vi "uService GUI.vi"(8 "error in (no error)":errorcluster, 11 "uService Template in":refnum<class "Tamer.lvclass">) -> (3 "uService Template out":refnum<class "Tamer.lvclass">)   [LabVIEW 2020, in "CIRCUS_uServices.lvlib" / "Tamer.lvlib" / "Tamer.lvclass"]
uses:
  Tamer.lvclass
  Tamer.lvclass/Tamer.ctl
  Link Chain GUI.ctl
  Monkey Summary.ctl
  TALOS/TALOS_PPL.lvlibp/Father of all uServices/Father of all uServices/Father of all uServices.lvclass
  TALOS/TALOS_PPL.lvlibp
  TALOS/TALOS_PPL.lvlibp/Guardian/Guardian/Requests.ctl
  TALOS/TALOS_PPL.lvlibp/Guardian/Guardian/Guardian.lvclass
  Run Utilities/TypeDefs/Monkey Status.ctl
  Run Utilities/Run Utilities.lvlib
  Stop Message.ctl
  C:/Users/marco/Documents/GitHub_Lab/CIRCUS/TALOS/TALOS_PPL.lvlibp/Father of all uServices/Father of all uServices/Father of all uServices.lvclass
  C:/Users/marco/Documents/GitHub_Lab/CIRCUS/TALOS/TALOS_PPL.lvlibp/Ancestor/Ancestor/Ancestor.lvclass
  C:/Users/marco/Documents/GitHub_Lab/CIRCUS/TALOS/Actor Framework.lvlibp/1abvi3w/vi.lib/ActorFramework/Actor/Actor.lvclass
  C:/Users/marco/Documents/GitHub_Lab/CIRCUS/CIRCUS uServices et al/Tamer/Tamer.lvclass
  Monkeys on display - picture.ctl
panel:
  in  "Pause":bool
  in  "Gracefully":bool=TRUE
  in  "Kill Process":bool
  in  "Skip Run":bool
  in  "Monkeys on display":T1
  in  "Tamer Picture":picture
  in  "Color 5":u32(colorbox)=16711680
  in  "Color 4":u32(colorbox)=8454019
  in  "Color 3":u32(colorbox)=16580480
  in  "Color 2":u32(colorbox)=8437759
  in  "Color":u32(colorbox)=16777225
  in  "Debug Mode":bool caption="Open the Debug\nWindow"
  out "Action History":string
  in  "Process":string(combo)
  out "The Stage":T2[][](array[typedef])
  in  "Rerun":bool
  in  "Stop Schedule":bool
  in  "stop New uService":bool
  in  "Reschedule":bool
  in  "Tamer Logo":picture
  # "The TAMER"
  # "Legend:"
  # "Stopped by an error"
  # "Finished well"
  # "Stopped by a user"
  # "Working"
  # "Pre-run init"
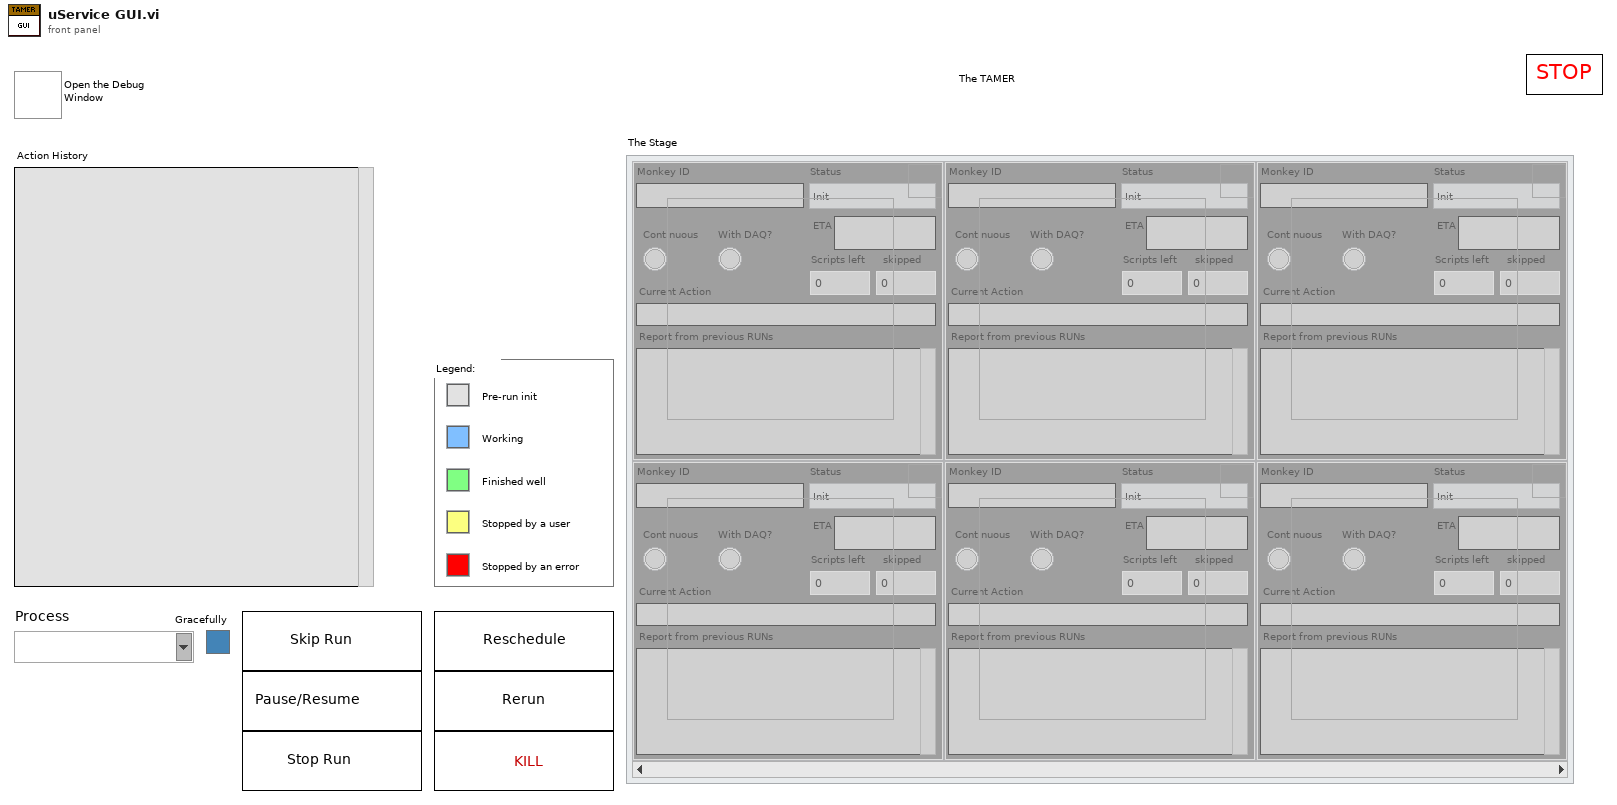
[diagram p1: front panel]
types:
  T1 = typedef "CIRCUS_uServices.lvlib/Tamer.lvlib/Tamer.lvclass/Monkeys on display - picture.ctl" = u16
  T2 = typedef "CIRCUS_uServices.lvlib/Tamer.lvlib/Tamer.lvclass/Monkey Summary.ctl" = cluster{"Color":u32, "Status":T3, "Continuous":bool, "Scripts left":u32, "Scripts skipped":u32, "ETA":string, "Current Action":string, "Report from previous RUNs":string, "Monkey ID":string, "With DAQ?":bool, "Linked?":T4, "Paused":bool}
  T3 = typedef "CIRCUS_uServices.lvlib/Run Utilities.lvlib/Monkey Status.ctl" = enum16{"Init", "Paused", "Ongoing", "Stopped", "Finished (no errors)", "Finished (with errors)"}
  T4 = typedef "CIRCUS_uServices.lvlib/Tamer.lvlib/Tamer.lvclass/Link Chain GUI.ctl" = bool
  T5 = typedef "CIRCUS_uServices.lvlib/Tamer.lvlib/Tamer.lvclass/Stop Message.ctl" = cluster{"Gracefully":bool, "Process":string}
  T6 = typedef "TALOS_PPL.lvlibp/Guardian.lvlib/Guardian.lvclass/Requests.ctl" = enum16{"Ready to Launch", "Start RUN", "Stop RUN", "Update DAQ Params", "Update Error Listbox", "Update Run Status", "Update Kasli Log", "Run Stopped with Errors", "Switch uS View"}
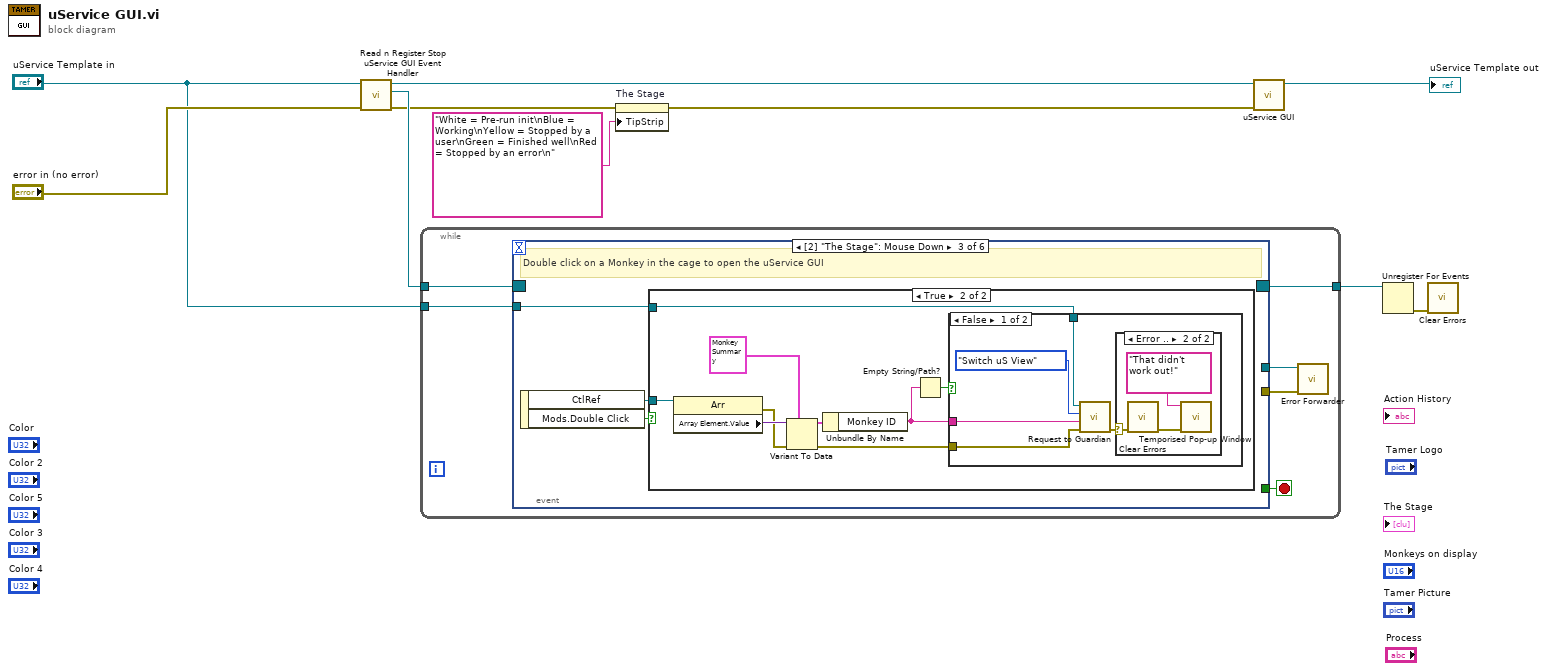
[diagram p0: block diagram]
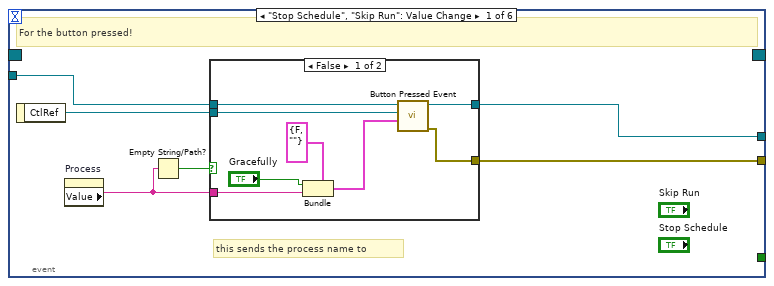
[diagram p2: hidden frame]
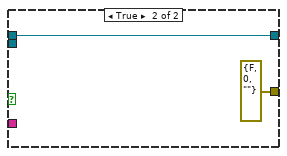
[diagram p3: hidden frame]
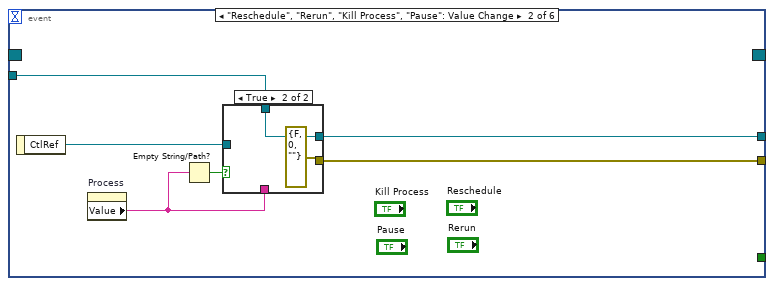
[diagram p4: hidden frame]
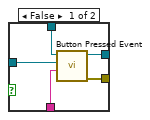
[diagram p5: hidden frame]
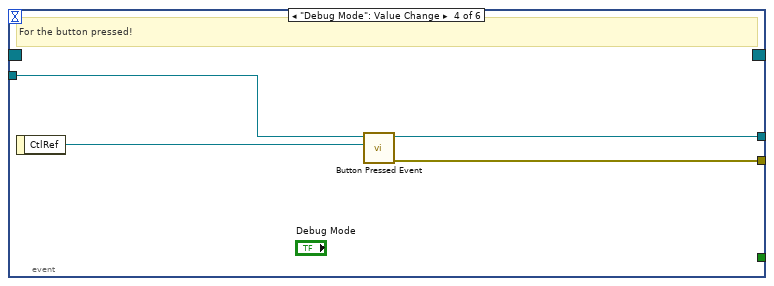
[diagram p9: hidden frame]
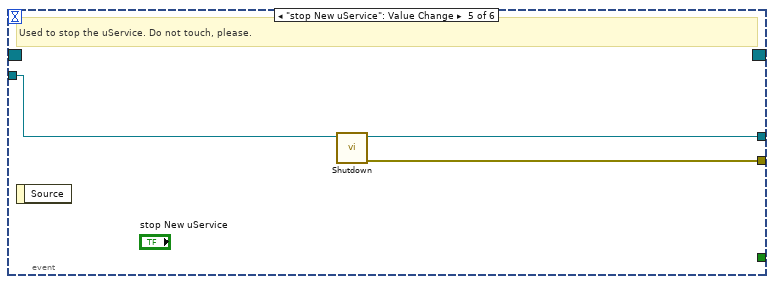
[diagram p10: hidden frame]
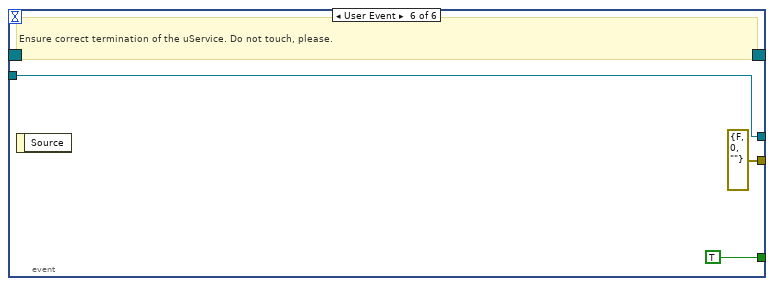
[diagram p11: hidden frame]
diagram:
  n1 = call-dynamic "Read n Register Stop uService GUI Event Handler .vi"("error in (no error)"="error in (no error)", "uService Template in"="uService Template in") -> ("error out"=w4:errorcluster, "Stop uService GUI Event Ref"=w8:refnum<event-registration>, "uService Template out"=w9:refnum<class "Tamer.lvclass">)  [unwired: 7 in]
  n2 = while {
    tunnel: [w16] -> w10
    tunnel: w8 -> [w14]
    tunnel: "uService Template in" -> [w13]
    stop <- w15 stop-if-true
    n3 = event shown="[2] \"The Stage\": Mouse Down" {
      selector: w14 -> [_ _ _ _ _ _]
      dyn-events: [_ _ _ _ _ _] -> w16
      timeout: _ -> [_ _ _ _ _ _]
      tunnel: [_ _ _ _ _ TRUE] -> w15
      tunnel: w13 -> [w22 w38 w47 w69 w72 w74]
      tunnel: [w17 w33 _ w67 w71 errorcluster {"status"=FALSE, "code"=0, "source"=""} ("error out")] -> w12
      tunnel: [w18 w34 _ w66 w70 w74] -> w11
      event "Stop Schedule", "Skip Run": Value Change {
        # "this sends the process name to"
        # "For the button pressed!"
        n4 = event-data() -> ("CtlRef"=w21:refnum<vi>)  [unwired: 1 in]
        n5 = property on="Process" class="CmbBox"() -> ("Value"=w19:string)  [unwired: 2 in, 2 out]
        n6 = Empty String/Path?(string/path=w19) -> (empty?=w20:bool)
        n7 = case shown="False" w20 {
          tunnel: w22 -> [w30 w32]
          tunnel: w21 -> [w29 _]
          tunnel: w19 -> [w27 _]
          tunnel: [w24 w32] -> w18
          tunnel: [w23 errorcluster {"status"=FALSE, "code"=0, "source"=""} ("error out")] -> w17
          frame False {
            n8 = Bundle(cluster=T5 {"Gracefully"=FALSE, "Process"=""}, "Gracefully"="Gracefully", "Process"=w27) -> (w26:T5)
            n9 = call-dynamic "Button Pressed Event.vi"("Data"=w26, "CtlRef"=w29, "uService Template in"=w30) -> ("error out"=w23:errorcluster, "uService Template out"=w24:refnum<class "Tamer.lvclass">)  [unwired: 7 in]
          }
          frame True {
          }
        }
      }
      event "Reschedule", "Rerun", "Kill Process", "Pause": Value Change {
        n10 = event-data() -> ("CtlRef"=w37:refnum<vi>)  [unwired: 1 in]
        n11 = property on="Process" class="CmbBox"() -> ("Value"=w35:string)  [unwired: 2 in, 2 out]
        n12 = Empty String/Path?(string/path=w35) -> (empty?=w36:bool)
        n13 = case shown="True" w36 {
          tunnel: w38 -> [w43 w45]
          tunnel: w37 -> [w42 _]
          tunnel: w35 -> [w41 _]
          tunnel: [w40 w45] -> w34
          tunnel: [w39 errorcluster {"status"=FALSE, "code"=0, "source"=""} ("error out")] -> w33
          frame False {
            n14 = call-dynamic "Button Pressed Event.vi"("Data"=w41, "CtlRef"=w42, "uService Template in"=w43) -> ("error out"=w39:errorcluster, "uService Template out"=w40:refnum<class "Tamer.lvclass">)  [unwired: 7 in]
          }
          frame True {
          }
        }
      }
      event "The Stage": Mouse Down {
        # "Double click on a Monkey in the cage to open the uService GUI"
        n15 = event-data() -> ("CtlRef"=w48:refnum<vi>, "Mods.Double Click"=w46:bool)  [unwired: 1 in]
        n16 = case shown="True" w46 {
          tunnel: w48 -> [_ w57]
          tunnel: w47 -> [_ w52]
          frame False {
            # "not a double click, ignore"
          }
          frame True {
            n17 = property class="Arr"(reference=w57) -> (error out=w55:errorcluster, "Array Element.Value"=w56:variant)  [unwired: 1 in, 1 out]
            n18 = Variant To Data(error in=w55, type=T2 {"Color"=8421504, "Status"=enum."Init", "Continuous"=FALSE, "Scripts left"=0, "Scripts skipped"=0, "ETA"="", "Current Action"="", "Report from previous RUNs"="", "Monkey ID"="", "With DAQ?"=FALSE, "Linked?"=FALSE, "Paused"=FALSE} ("Monkey Summary"), Variant=w56) -> (data=w53:T2, error out=w51:errorcluster)
            n19 = Unbundle By Name(w53) -> ("Monkey ID"=w49:string)
            n20 = Empty String/Path?(string/path=w49) -> (empty?=w50:bool)
            n21 = case shown="False" w50 {
              tunnel: w49 -> [w61 _]
              tunnel: w52 -> [w60 _]
              tunnel: w51 -> [w58 _]
              frame False {
                n22 = call "Request to Guardian.vi"("error in (no error)"=w58, "Data"=w61, "Requests"=Requests."Switch uS View", "Father of all uServices in"=w60) -> ("error out"=w59:errorcluster)  [unwired: 6 in, 1 out]
                n23 = case shown="Error .." w59 {
                  selector: w59 -> [_ w65]
                  frame No Error {
                  }
                  frame Error {
                    n24 = call <vilib>:"Clear Errors.vi"("error in (no error)"=w65) -> ("error out"=w64:errorcluster)  [unwired: 5 in, 1 out]
                    n25 = call "Temporised Pop-up Window.vi"("error in (no error)"=w64, "Text"="That didn't work out!") -> ()  [unwired: 9 in, 1 out]
                  }
                }
              }
              frame True {
                # "empty ID, ignore"
              }
            }
          }
        }
      }
      event "Debug Mode": Value Change {
        # "For the button pressed!"
        n26 = event-data() -> ("CtlRef"=w68:refnum<vi>)  [unwired: 1 in]
        n27 = call-dynamic "Button Pressed Event.vi"("CtlRef"=w68, "uService Template in"=w69) -> ("error out"=w67:errorcluster, "uService Template out"=w66:refnum<class "Tamer.lvclass">)  [unwired: 8 in]
      }
      event "stop New uService": Value Change {
        # "Used to stop the uService. Do not touch, please."
        n28 = event-data() -> ()  [unwired: 1 in, 1 out]
        n29 = call "Shutdown.vi"("Father of all uServices in"=w72) -> ("error out"=w71:errorcluster, "Father of all uServices out"=w70:refnum<class "Tamer.lvclass">)  [unwired: 9 in]
      }
      event User Event {
        # "Ensure correct termination of the uService. Do not touch, please."
        n30 = event-data() -> ()  [unwired: 1 in, 1 out]
      }
    }
    n31 = call "Error Forwarder.vi"("error in (no error)"=w12, "Father of all uServices in"=w11) -> ()  [unwired: 10 in]
  }
  n32 = property on="The Stage" class="Arr"(error in=w4, "TipStrip"="White = Pre-run init\nBlue = Working\nYellow = Stopped by a user\nGreen = Finished well\nRed = Stopped by an error\n" ("Tip Strip")) -> (error out=w2:errorcluster)  [unwired: 1 in, 1 out]
  n33 = call-parent "uService GUI.vi"("error in (no error)"=w2, "uService Template in"=w9) -> ("uService Template out"=→"uService Template out":refnum<class "Tamer.lvclass">)  [unwired: 9 in]
  n34 = Unregister For Events(event registration refnum=w10) -> (error out=w1:errorcluster)  [unwired: 1 in]
  n35 = call <vilib>:"Clear Errors.vi"("error in (no error)"=w1) -> ()  [unwired: 5 in, 2 out]
